vi "Memory.Pointer.Read (safe).vi"(8 "error in (no error)":errorcluster, 9 "offset (0)":u64 format="%d bytes", 10 "length (-1: all)":i64=-1 format="%d bytes", 11 "Pointer in":refnum<class "Memory.Pointer.lvclass">) -> (0 "error out":errorcluster, 1 "offset dup":u64 format="%d bytes", 2 "data":string, 3 "Pointer out":refnum<class "Memory.Pointer.lvclass">)   [LabVIEW 2016, in "LabVIEW Memory Manager.lvlib" / "Memory.Pointer.lvclass"]
uses:
  Memory.Pointer.lvclass
  Memory.Pointer.lvclass/Memory.Pointer.ctl
  Accessors/Memory.Pointer.Get Address.vi
  LabVIEW Memory Manager.lvlib
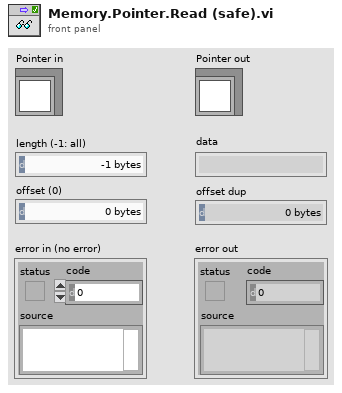
[diagram p1: front panel]
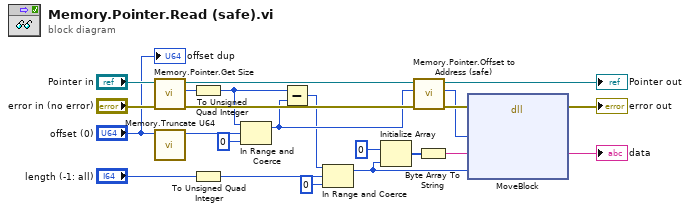
[diagram p0: block diagram]
diagram:
  n1 = call "Memory.Pointer.Get Size.vi"("error in (no error)"="error in (no error)", "Pointer in"="Pointer in") -> ("error out"=w17:errorcluster, "size"=w8:i64, "Pointer out"=w18:refnum<class "Memory.Pointer.lvclass">)  [unwired: 7 in]
  n2 = call "Memory.Truncate U64.vi"("U64"="offset (0)") -> ("truncated U64"=w2:u64)  [unwired: 10 in]
  n3 = To Unsigned Quad Integer(1:w8) -> (0:w7:u64)
  n4 = To Unsigned Quad Integer(1:"length (-1: all)") -> (0:w3:u64)
  n5 = In Range and Coerce(upper limit=w7, x=w2, lower limit=u64 0) -> (coerced(x)=w5:u64)  [unwired: 1 out]
  n6 = Subtract(x=w7, y=w5) -> (x-y=w4:u64)
  n7 = In Range and Coerce(upper limit=w4, x=w3, lower limit=u64 0) -> (coerced(x)=w16:u64)  [unwired: 1 out]
  n8 = Initialize Array(u8 0 ("element"), w16) -> (w13:u8[])
  n9 = call "Memory.Pointer.Offset to Address (safe).vi"("error in (no error)"=w17, "offset"=w5, "Pointer in"=w18) -> ("error out"=w11:errorcluster, "address"=w10:u64, "Pointer out"=→"Pointer out":refnum<class "Memory.Pointer.lvclass">)  [unwired: 5 in, 1 out]
  n10 = Byte Array To String(unsigned byte array=w13) -> (string=w12:string)
  n11 = dll-call lib="LabVIEW" fn="MoveBlock"(error in=w11, "src pointer"=w10, "dst pointer"=w12, "size"=w16) -> (error out=→"error out":errorcluster, "dst pointer"=→"data":string)  [unwired: 5 in, 1 out]
  "offset dup" <- "offset (0)"
